vi "motor test.vi"() -> ()   [LabVIEW 2012]
uses:
  <vilib>/rvi/interface/nirviOpenFPGA/nirviOpenFPGA.xnode
  <vilib>/robotics/Navigation/shared/WorldMap/OccupancyGridWorldMap/NI_Robotics_OccupancyGridWorldMap.lvclass
  <vilib>/rvi/interface/nirviCloseFPGA/nirviCloseFPGA.xnode
  <vilib>/rvi/interface/nirviReadWriteControl/nirviReadWriteControl.xnode
  <vilib>/Platform/TimedLoop/XDataNode/wakeup.ctl
  <vilib>/Platform/TimedLoop/XDataNode/XDNodeRunTimeDep.lvlib
  <vilib>/Platform/TimedLoop/XDataNode/nitl_modes.ctl
  <vilib>/Platform/TimedLoop/XDataNode/timing_clust.ctl
  <vilib>/Platform/TimedLoop/XDataNode/XDataNode.xnode
  Compass/Compass IO.lvlib
  Mouse IO/Mouse IO.lvlib
  FPGA Bitfiles/NIARCDemo-kyle_FPGATarget_FPGAToplevel_9c4As6+H2cU.lvbitx
  <vilib>/FPGAPlugInAG/sbRIO-9636/niLvFpga_Open_sbRIO-9636.vi
  <vilib>/rvi/interface/common/dynamic/niFpgaDynamicAddResources.vi
  <vilib>/FPGAPlugInAG/Dynamic/niLvFpga_Close_Dynamic.vi
  NiFpgaLv.dll
  <vilib>/Utility/error.llb/Error Cluster From Error Code.vi
  <vilib>/rvi/interface/Simulation/niFpgaSimulationCallBeginRW.vi
  <vilib>/rvi/errors/niLvFpgaAdjustHostInterfaceError.vi
panel:
  out "Object Avoid?":bool
  in  "OK Button":bool
  in  "clockwise":bool
  in  "Anit clockwise":bool
  in  "Speed":dbl
  in  "Left":bool
  in  "Right":bool
  in  "Bck":bool
  in  "Fwrd":bool
  in  "Deg ofset":dbl
  out "Y Pos":i32
  out "X Pos":i32
  in  "Grid Draw":i16=100
  out "Intensity Graph":dbl[][](graph)
  out "Motor y out":dbl
  out "Motor x out":dbl
  in  "Array":i16[](array[numeric])
  in  "Waypoint":i16
  in  "Speed":dbl
  out "Distance left":dbl
  out "Distance right":dbl
  in  "Enable":bool
  in  "x start":i32=1
  in  "y start":i32=1
  out "X dispacement":i32
  out "Y displacement":i32
  out "Rotation (deg)":dbl
  out "Distance mid":dbl
  out "Finished late":bool
  in  "stop 2":bool
  in  "Boolean":bool
  in  "Manual control":bool
  in  "stop":bool
  # "Motor Control"
  # "Mapping"
  # "Waypoints"
  # "x"
  # "y"
  # "x start"
  # "y start"
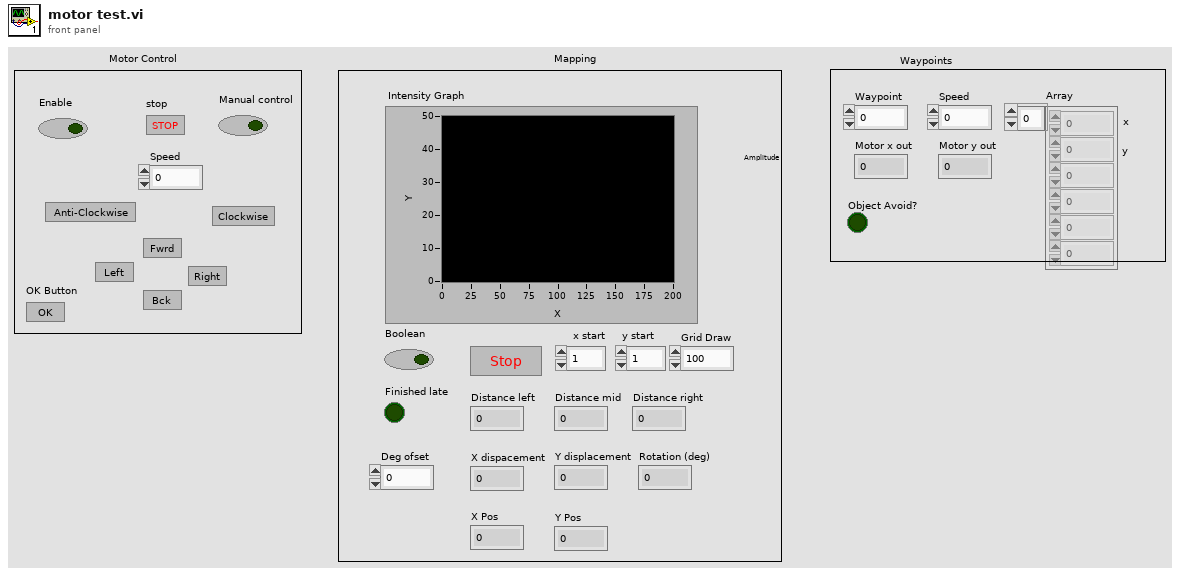
[diagram p1: front panel]
types:
  T1 = cluster{"FPGA VI Reference":refnum<k20>, "Timeout":i32}
  T2 = typedef "XDNodeRunTimeDep.lvlib/timing_clust.ctl" = cluster{"Expected End [f-1]":u64, "Actual End [f-1]":u64, "Finished Late? [f-1]":bool, "Expected End [i-1]":u64, "Actual End [i-1]":u64, "Finished Late? [i-1]":bool, "Expected Start [i]":u64, "Actual Start [i]":u64, "Expected Start [f]":u64, "Actual Start [f]":u64, "Source Name":string, "Structure Name":string, "Period":i64, "Deadline":i64, "Offset":i64, "Start":i64, "Priority":i32, "Timeout":i32, "Mode":T3, "Wakeup Reason":T4, "Error":errorcluster, "Source Type":string, "Secondary Source Type":string, "Global End Time":u64, "Global Start Time":u64, "Frame Duration":u64, "Iteration Duration":u64, "Assigned CPU":i32, "I/O Scan Engine Mode":u32}
  T3 = typedef "XDNodeRunTimeDep.lvlib/nitl_modes.ctl" = enum32{"No Change", "Process missed periods, maintain original phase", "Discard missed periods, maintain original phase", "Process missed periods, ignore original phase", "Discard missed periods, ignore original phase"}
  T4 = typedef "XDNodeRunTimeDep.lvlib/wakeup.ctl" = enum32{"Normal", "Aborted", "Asynchronous wakeup", "Timing source error", "Timed loop error", "Timeout"}
  T5 = cluster{"FPGA VI Reference":refnum<k20>, "Port Number":u8}
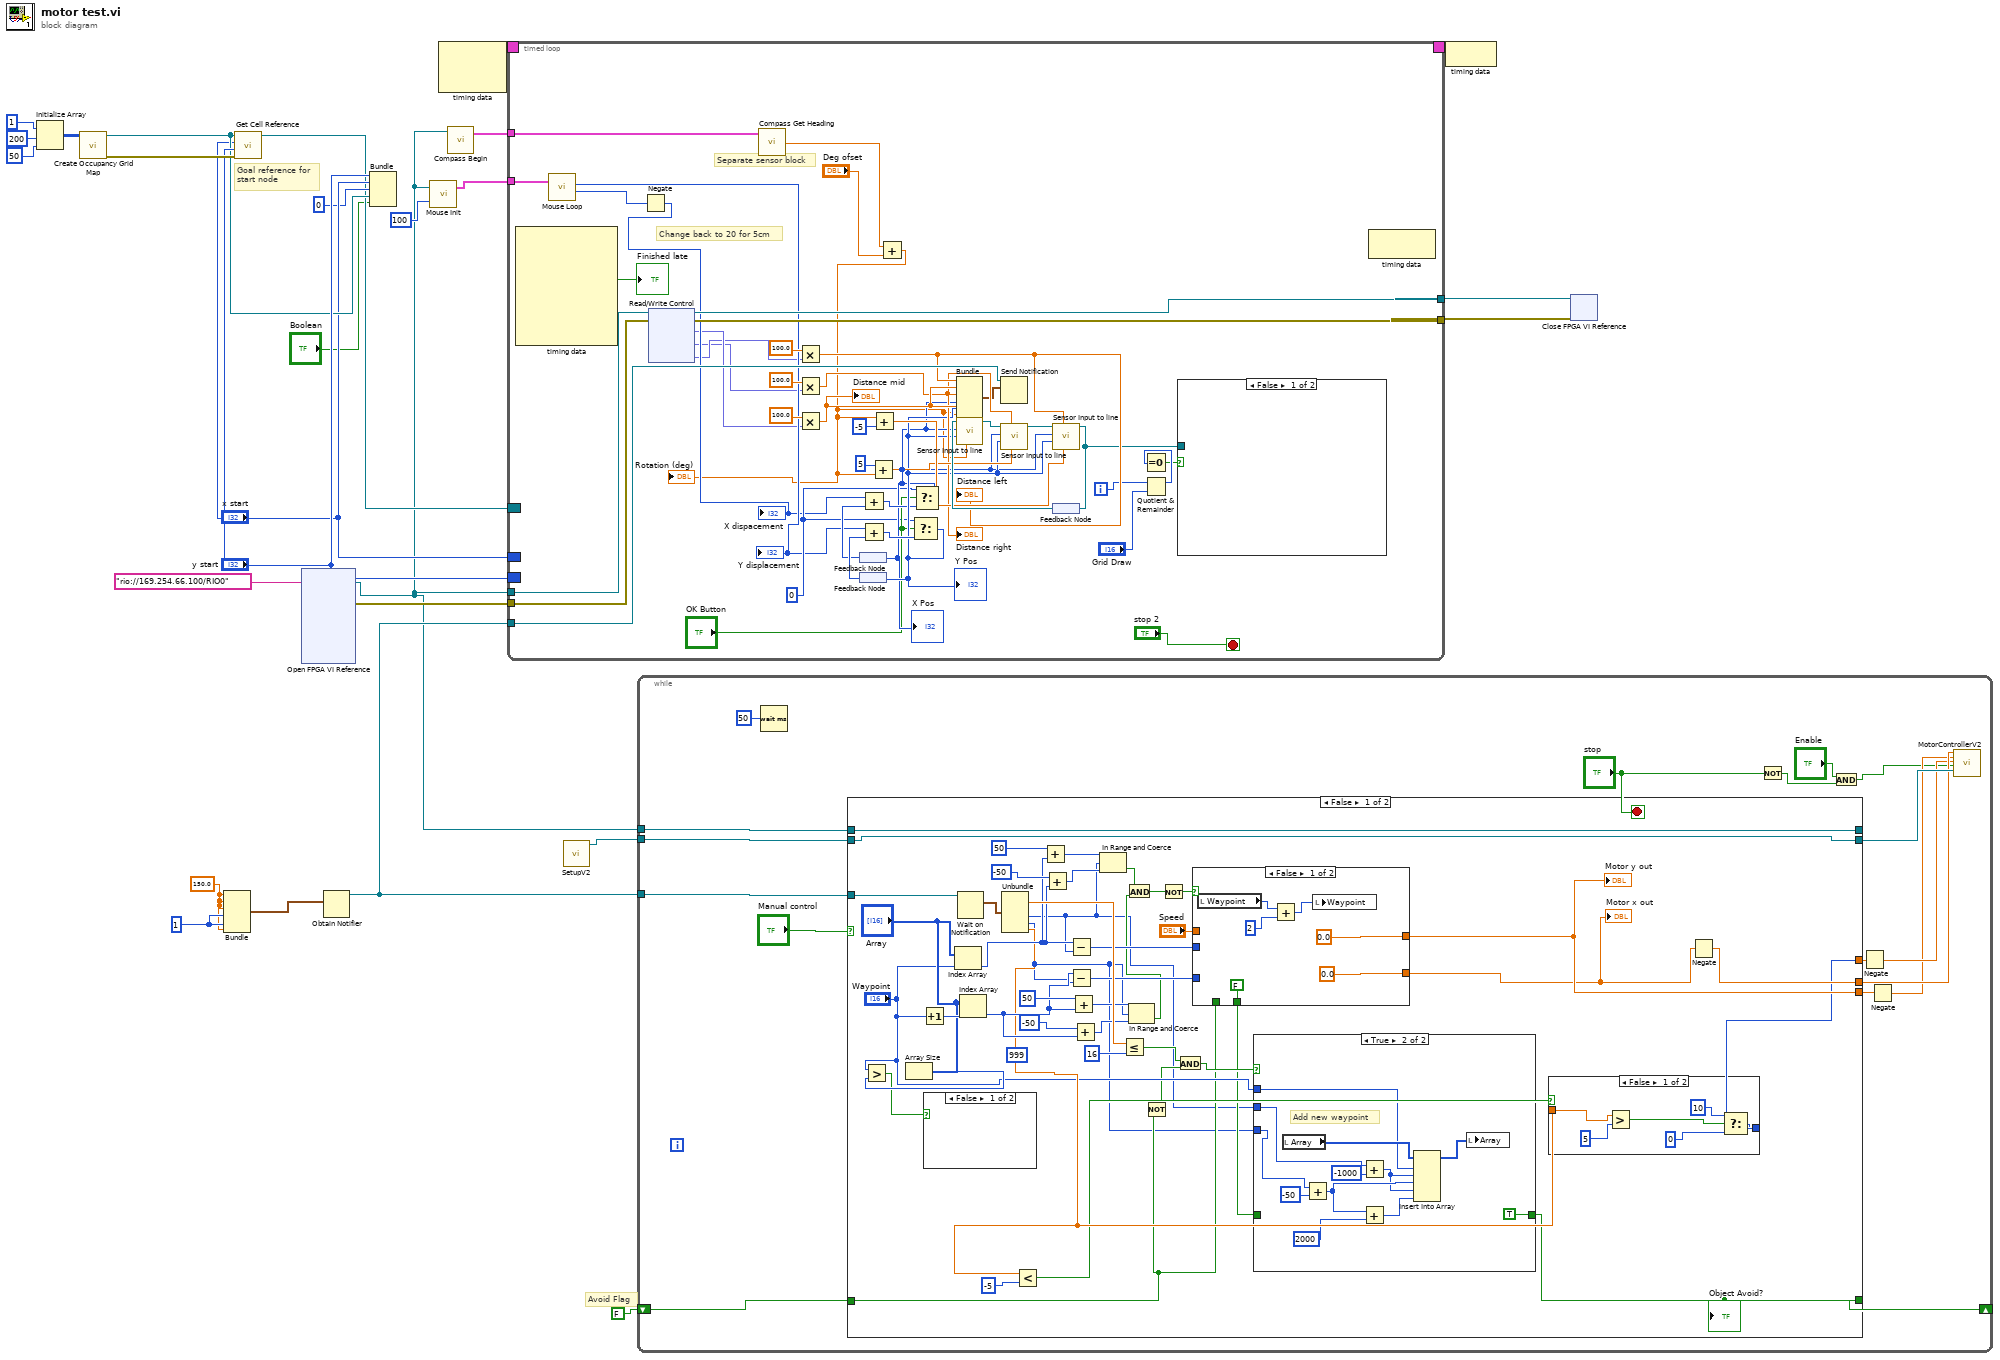
[diagram p0: block diagram]
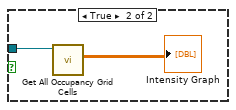
[diagram p2: hidden frame]
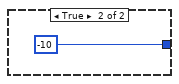
[diagram p4: hidden frame]
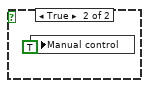
[diagram p5: hidden frame]
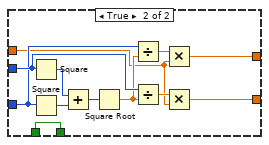
[diagram p6: hidden frame]
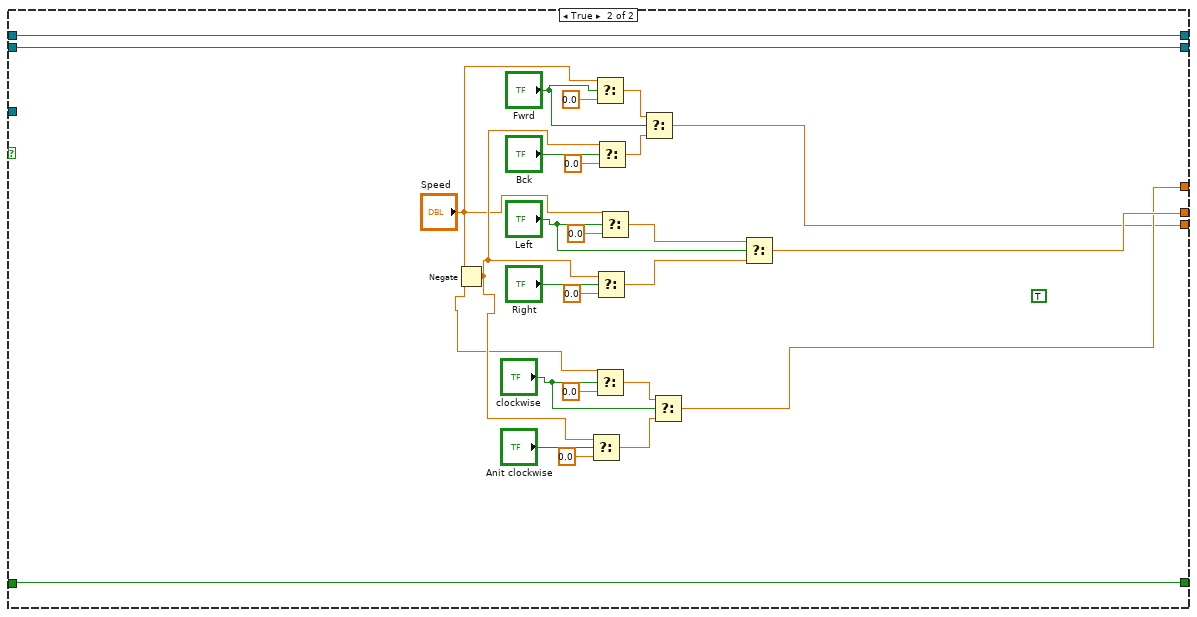
[diagram p7: hidden frame]
diagram:
  w5 = 1
  w3 = 150.0
  # "Avoid Flag"
  # "Separate sensor block"
  # "Goal reference for\nstart node"
  n1 = Initialize Array(1, 200, 50) -> (w13:i32[][])
  n2 = call <vilib>:"Create Occupancy Grid Map.vi"("occupancy grid"=w13) -> ("error out"=w25:errorcluster, "map reference out"=w23:refnum<data-value>)  [unwired: 9 in]
  n3 = Bundle(w3, w3, w3, w5, w5, w3) -> (w10:cluster{dbl, dbl, dbl, i32, i32, dbl})  [unwired: 1 in]
  n4 = call <vilib>:"Get Cell Reference.vi"("error in (no error)"=w25, "y"="y start", "x"="x start", "map reference in"=w23) -> ("map reference out"=w12:refnum<data-value>)  [unwired: 4 in, 3 out]
  n5 = xnode "Open FPGA VI Reference"("resource name"=tag "rio://169.254.66.100/RIO0") -> ("FPGA VI Reference Out"=w1:refnum<k20>, "error out"=w17:errorcluster)  [unwired: 1 in]
  n6 = Obtain Notifier(notification data type=w10) -> (notifier out=w9:refnum<notifier>)  [unwired: 3 in, 2 out]
  n7 = Bundle("y start"="y start", "x start"="x start", 0, "map reference out"=w23, "Boolean"="Boolean") -> ()  [unwired: 1 in, 1 out]
  n8 = call "Mouse Init.vi"("Timeout (ms)"=100, "FPGA VI Reference In"=w1) -> ("Mouse Sensor"=w7:T1)  [unwired: 1 out]
  n9 = node-c288() -> (w27:T2)  [unwired: 2 in]
  n10 = call "Compass Begin.vi"("FPGA VI Reference"=w1) -> ("FPGA Information Out"=w8:T5)  [unwired: 3 in, 1 out]
  n11 = timed-loop {
    border: "y start" -> [_]
    border: "x start" -> [_]
    border: w12 -> [_]
    tunnel: [w69] -> w20
    tunnel: [w68] -> w19
    timing: w27 -> [_]
    timing-out: [_] -> w26
    tunnel: w1 -> [w66]
    tunnel: w17 -> [w65]
    tunnel: w9 -> [w56]
    tunnel: w8 -> [w48]
    tunnel: w7 -> [w47]
    i -> [w46]
    stop <- "stop 2" stop-if-true
    w35 = 0
    # "Change back to 20 for 5cm"
    n12 = node-c288() -> (→"Finished late":bool)  [unwired: 1 in, 7 out]
    n13 = call "Mouse Loop.vi"("Mouse Sensor In"=w47) -> ("x displacement"=w34:i8, "y displacement"=w33:i8)  [unwired: 2 in, 1 out]
    "Y displacement" <- w34
    n14 = Negate(x=w33) -> (-x=w32:i8)
    "X dispacement" <- w32
    n15 = xnode "Read/Write Control"("FPGA VI Reference In"=w66, "error in"=w65) -> ("FPGA VI Reference Out"=w69:refnum<k20>, "error out"=w68:errorcluster, "IR 0"=w30:fxp<+/-,24,5>, "IR 1"=w28:fxp<+/-,24,5>, "IR 2"=w29:fxp<+/-,24,5>)
    n16 = call "Compass Get Heading.vi"("FPGA Information In"=w48) -> ("Heading (deg)"=w42:dbl)  [unwired: 1 in, 2 out]
    n17 = Multiply(x=100.0, y=w29) -> (x*y=w53:dbl)
    "Distance left" <- w53
    n18 = Multiply(x=100.0, y=w28) -> (x*y=w51:dbl)
    "Distance right" <- w51
    n19 = Multiply(x=100.0, y=w30) -> (x*y=w52:dbl)
    "Distance mid" <- w52
    n20 = feedback #1() -> (w71:i32)
    n21 = feedback #2() -> (w72:i32)
    n22 = Add(x=w32, y=w71) -> (x+y=w38:i32)
    n23 = Add(x=w34, y=w72) -> (x+y=w40:i32)
    n24 = Add(x=w42, y="Deg ofset") -> (x+y=w31:dbl)
    "Rotation (deg)" <- w31
    n25 = Add(x=5, y=w31) -> (x+y=w54:dbl)
    n26 = Add(x=w31, y=-5) -> (x+y=w55:dbl)
    n27 = Select(t=w35, s="OK Button", f=w40) -> (s? t:f=w39:i32)
    "Y Pos" <- w39
    n28 = feedback-in #2(w39) -> ()
    n29 = Select(t=w35, s="OK Button", f=w38) -> (s? t:f=w37:i32)
    "X Pos" <- w37
    n30 = feedback-in #1(w37) -> ()
    n31 = Bundle(w53, w52, w51, w37, w39, w31) -> (w50:cluster{dbl, dbl, dbl, i32, i32, dbl})  [unwired: 1 in]
    n32 = Send Notification(notification=w50, notifier=w56) -> ()  [unwired: 1 in, 2 out]
    n33 = feedback #3() -> (w70:refnum<data-value>)
    n34 = call "Sensor Input to line.vi"("Degrees"=w31, "distance front"=w52, "sensor y"=w39, "Sensor x"=w37, "map reference in"=w70) -> ("map reference out 2"=w63:refnum<data-value>)  [unwired: 5 in, 1 out]
    n35 = call "Sensor Input to line.vi"("Degrees"=w54, "distance front"=w51, "sensor y"=w39, "Sensor x"=w37, "map reference in"=w63) -> ("map reference out 2"=w62:refnum<data-value>)  [unwired: 5 in, 1 out]
    n36 = call "Sensor Input to line.vi"("Degrees"=w55, "distance front"=w53, "sensor y"=w39, "Sensor x"=w37, "map reference in"=w62) -> ("map reference out 2"=w49:refnum<data-value>)  [unwired: 5 in, 1 out]
    n37 = feedback-in #3(w49) -> ()
    n38 = Quotient & Remainder(x=w46, y="Grid Draw") -> (x-y*floor(x/y)=w44:i32)  [unwired: 1 out]
    n39 = Equal To 0?(x=w44) -> (x = 0?=w43:bool)
    n40 = case shown="False" w43 {
      tunnel: w49 -> [_ w74]
      frame False {
      }
      frame True {
        n41 = call <vilib>:"Get All Occupancy Grid Cells.vi"("map reference in"=w74) -> ("occupancy grid"=→"Intensity Graph":dbl[][])  [unwired: 8 in, 2 out]
      }
    }
    n42 = node-c288() -> ()  [unwired: 1 in, 1 out]
  }
  n43 = call "SetupV2.vi"() -> ("mecanum steering frame out"=w4:refnum<class "NI_Robotics_Mecanum Steering Frame.lvclass">)  [unwired: 10 in, 1 out]
  n44 = while {
    tunnel: w4 -> [w94]
    tunnel: w1 -> [w93]
    tunnel: w9 -> [w87]
    shift-right: [w78] -> _
    shift-left: FALSE -> [w79]
    stop <- "stop" stop-if-true
    n45 = Wait (ms)(milliseconds to wait=50) -> ()  [unwired: 1 out]
    n46 = case shown="False" "Manual control" {
      tunnel: w94 -> [w134 w201]
      tunnel: w93 -> [w135 w202]
      tunnel: [w135 w202] -> _
      tunnel: [w125 w180] -> w85
      tunnel: [w104 w179] -> w84
      tunnel: [w129 w178] -> w82
      tunnel: [w134 w201] -> w86
      tunnel: w87 -> [w137 _]
      tunnel: w79 -> [w99 w177]
      tunnel: [w100 w177] -> w78
      frame False {
        (unwired) 999
        n47 = Array Size(array="Array") -> (size(s)=w123:i32)
        n48 = Greater?(x="Waypoint", y=w123) -> (0:w122:bool)
        n49 = Increment(x="Waypoint") -> (x+1=w130:i16)
        n50 = case shown="False" w122 {
          frame False {
          }
          frame True {
            n51 = local write "Manual control"(TRUE) -> ()
          }
        }
        n52 = Index Array(array="Array", index="Waypoint") -> (element=w117:i16)
        n53 = Wait on Notification(notifier=w137) -> (notification=w136:cluster{dbl, dbl, dbl, i32, i32, dbl})  [unwired: 3 in, 3 out]
        n54 = Index Array(array="Array", index=w130) -> (element=w109:i16)
        n55 = Unbundle(w136) -> (w128:dbl, w96:i32, w95:i32, w107:dbl)  [unwired: 2 out]
        n56 = Less?(x=w107, y=-5) -> (x < y?=w105:bool)
        n57 = Add(x=50, y=w117) -> (x+y=w118:i32)
        n58 = Add(x=-50, y=w117) -> (x+y=w120:i32)
        n59 = Subtract(x=w117, y=w96) -> (x-y=w121:i32)
        n60 = Subtract(x=w109, y=w95) -> (x-y=w110:i32)
        n61 = Add(x=50, y=w109) -> (x+y=w112:i32)
        n62 = Add(x=-50, y=w109) -> (x+y=w114:i32)
        n63 = In Range and Coerce(upper limit=w118, x=w96, lower limit=w120) -> (In Range?=w115:bool)  [unwired: 1 out]
        n64 = Less Or Equal?(x=w128, y=16) -> (x <= y?=w103:bool)
        n65 = In Range and Coerce(upper limit=w112, x=w95, lower limit=w114) -> (In Range?=w108:bool)  [unwired: 1 out]
        n66 = And(x=w115, y=w108) -> (x .and. y?=w133:bool)
        n67 = Not(x=w99) -> (.not. x?=w97:bool)
        n68 = Not(x=w133) -> (.not. x?=w132:bool)
        n69 = And(x=w103, y=w97) -> (x .and. y?=w101:bool)
        n70 = case shown="False" w132 {
          tunnel: w121 -> [_ w173]
          tunnel: w110 -> [_ w171]
          tunnel: "Speed" -> [_ w168]
          tunnel: [0.0 w167] -> w126
          tunnel: [0.0 w166] -> w129
          tunnel: w99 -> [_ w165]
          tunnel: [FALSE w165] -> w98
          frame False {
            n71 = local read "Waypoint"() -> (w162:i16)
            n72 = Add(x=w162, y=2) -> (x+y=w160:i32)
            n73 = local write "Waypoint"(w160) -> ()
          }
          frame True {
            n74 = Square(x=w173) -> (x^2=w175:i32)
            n75 = Square(x=w171) -> (x^2=w176:i32)
            n76 = Add(x=w175, y=w176) -> (x+y=w174:i32)
            n77 = Square Root(x=w174) -> (sqrt(x)=w172:dbl)
            n78 = Divide(x=w171, y=w172) -> (x/y=w169:dbl)
            n79 = Divide(x=w173, y=w172) -> (x/y=w170:dbl)
            n80 = Multiply(x=w169, y=w168) -> (x*y=w166:dbl)
            n81 = Multiply(x=w170, y=w168) -> (x*y=w167:dbl)
          }
        }
        "Motor x out" <- w126
        "Motor y out" <- w129
        n82 = case shown="True" w101 {
          tunnel: "Waypoint" -> [_ w149]
          tunnel: w95 -> [_ w147]
          tunnel: w96 -> [_ w145]
          tunnel: w98 -> [w138 _]
          tunnel: [w138 TRUE] -> w100
          frame False {
          }
          frame True {
            # "Add new waypoint"
            n83 = local read "Array"() -> (w150:i16[])
            n84 = Add(x=w147, y=-50) -> (x+y=w141:i32)
            n85 = Add(x=w145, y=-1000) -> (x+y=w139:i32)
            n86 = Add(x=w141, y=2000) -> (x+y=w140:i32)
            n87 = Insert Into Array(array=w150, index=w149, new element #1=w139, new element #2=w141, new element #3=w139, new element #4=w140) -> (w144:i16[])
            n88 = local write "Array"(w144) -> ()
          }
        }
        "Object Avoid?" <- w100
        n89 = case shown="False" w105 {
          tunnel: w107 -> [w154 _]
          tunnel: [w152 -10] -> w104
          frame False {
            n90 = Greater?(x=w154, y=5) -> (0:w155:bool)
            n91 = Select(t=10, s=w155, f=0) -> (s? t:f=w152:i32)
          }
          frame True {
          }
        }
        n92 = Negate(x=w126) -> (-x=w125:dbl)
      }
      frame True {
        (unwired) TRUE
        n93 = Negate(x="Speed") -> (-x=w184:dbl)
        n94 = Select(t=w184, s="Anit clockwise", f=0.0) -> (s? t:f=w188:dbl)
        n95 = Select(t="Speed", s="Fwrd", f=0.0) -> (s? t:f=w198:dbl)
        n96 = Select(t="Speed", s="clockwise", f=0.0) -> (s? t:f=w187:dbl)
        n97 = Select(t=w184, s="Right", f=0.0) -> (s? t:f=w196:dbl)
        n98 = Select(t=w184, s="Bck", f=0.0) -> (s? t:f=w199:dbl)
        n99 = Select(t="Speed", s="Left", f=0.0) -> (s? t:f=w195:dbl)
        n100 = Select(t=w198, s="Fwrd", f=w199) -> (s? t:f=w178:dbl)
        n101 = Select(t=w187, s="clockwise", f=w188) -> (s? t:f=w179:dbl)
        n102 = Select(t=w195, s="Left", f=w196) -> (s? t:f=w180:dbl)
      }
    }
    n103 = Not(x="stop") -> (.not. x?=w90:bool)
    n104 = And(x="Enable", y=w90) -> (x .and. y?=w80:bool)
    n105 = Negate(x=w84) -> (-x=w83:dbl)
    n106 = Negate(x=w82) -> (-x=w81:dbl)
    n107 = call "MotorControllerV2.vi"("X Velocity (m/s)"=w85, "Y Velocity (m/s)"=w81, "Angular Velocity (rad/s)"=w83, "Enable"=w80, "mecanum steering frame in"=w86) -> ()  [unwired: 13 in, 2 out]
  }
  n108 = node-c288(w26) -> ()
  n109 = xnode "Close FPGA VI Reference"("FPGA VI Reference In"=w20, "error in"=w19) -> ()  [unwired: 1 out]
